vi "Statistical measure - basics percentual - 1.vi"(5 "Data measured":dbl[](array[numeric]), 9 "Data reference":dbl[](array[numeric])) -> (3 "x != y?":bool, 8 "Statistcs":T1 {"mean meas" format="%.10f"; "min meas" format="%.10f"; "max meas" format="%.10f"; "mean dev" format="%.10f"; "min dev" format="%.10f"; "max dev" format="%.10f"; "mean ref" format="%.10f"; "min ref" format="%.10f"; "max ref" format="%.10f"})   [LabVIEW 2019]
panel:
  # "Statistical Measure - basics percentual - 1"
  # "array size"
  # "Deviaton"
  # "Measured"
  # "Reference"
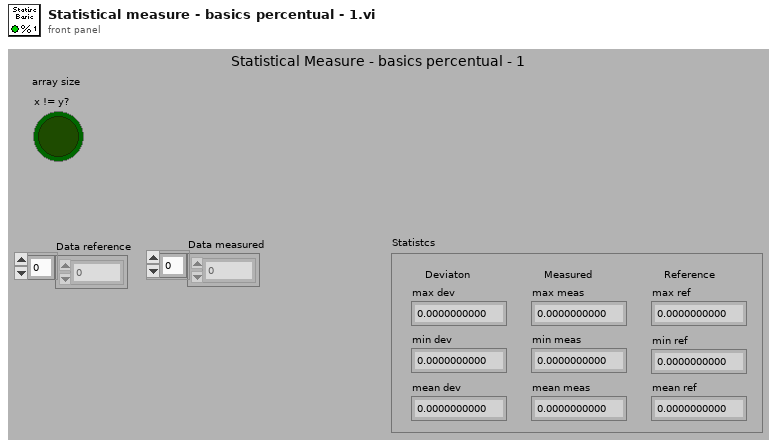
[diagram p1: front panel]
types:
  T1 = cluster{"max ref":dbl, "min ref":dbl, "mean ref":dbl, "max dev":dbl, "min dev":dbl, "mean dev":dbl, "max meas":dbl, "min meas":dbl, "mean meas":dbl}
  T2 = cluster{dbl, dbl, dbl, dbl, dbl, dbl, dbl, dbl, dbl}
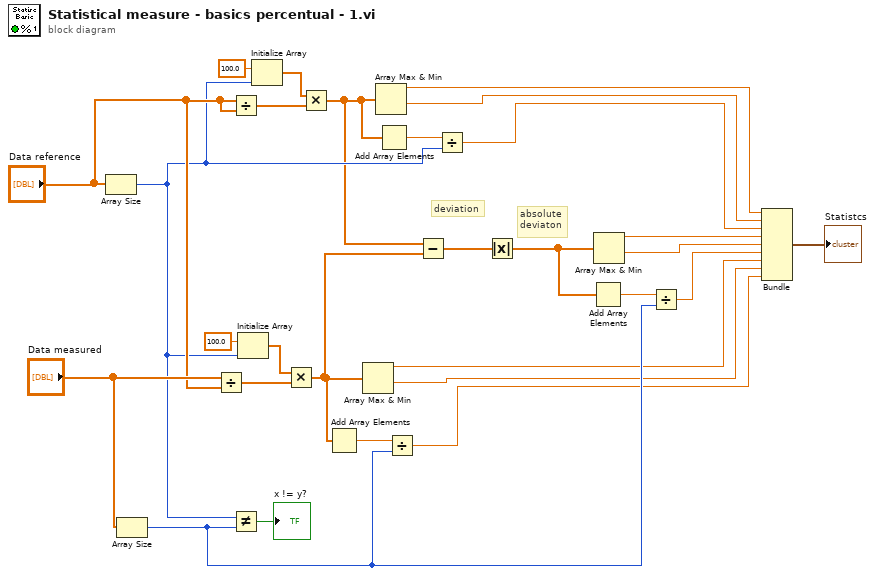
[diagram p0: block diagram]
diagram:
  # "deviation"
  # "absolute\ndeviaton"
  n1 = Array Size(array="Data reference") -> (size(s)=w3:i32)
  n2 = Array Size(array="Data measured") -> (size(s)=w23:i32)
  n3 = Divide(x="Data measured", y="Data reference") -> (x/y=w10:dbl[])
  n4 = Divide(x="Data reference", y="Data reference") -> (x/y=w7:dbl[])
  n5 = Not Equal?(x=w3, y=w23) -> (x != y?=→"x != y?":bool)
  n6 = Initialize Array(100.0 ("element"), w3) -> (w8:dbl[])
  n7 = Initialize Array(100.0 ("element"), w3) -> (w4:dbl[])
  n8 = Multiply(x=w8, y=w10) -> (x*y=w1:dbl[])
  n9 = Multiply(x=w4, y=w7) -> (x*y=w2:dbl[])
  n10 = Add Array Elements(numeric array=w1) -> (sum=w24:dbl)
  n11 = Array Max & Min(array=w1) -> (max value=w14:dbl, min value=w13:dbl)  [unwired: 2 out]
  n12 = Array Max & Min(array=w2) -> (max value=w20:dbl, min value=w19:dbl)  [unwired: 2 out]
  n13 = Add Array Elements(numeric array=w2) -> (sum=w22:dbl)
  n14 = Divide(x=w24, y=w23) -> (x/y=w12:dbl)
  n15 = Subtract(x=w2, y=w1) -> (x-y=w28:dbl[])
  n16 = Divide(x=w22, y=w3) -> (x/y=w18:dbl)
  n17 = Absolute Value(x=w28) -> (abs(x)=w26:dbl[])
  n18 = Add Array Elements(numeric array=w26) -> (sum=w25:dbl)
  n19 = Array Max & Min(array=w26) -> (max value=w17:dbl, min value=w16:dbl)  [unwired: 2 out]
  n20 = Divide(x=w25, y=w23) -> (x/y=w15:dbl)
  n21 = Bundle(w20, w19, w18, w17, w16, w15, w14, w13, w12) -> (→"Statistcs":T2)  [unwired: 1 in]
